vi "Section Names.vi"() -> (0 "Cluster":cluster{"Motion Settings":string}={"Motion Settings"="Motion Settings"})   [LabVIEW 2016, in "Hardware.lvlib" / "Motions.lvlib" / "Motions Configuration.lvclass"]
uses:
  <userlib>/Common Components/Hardware/Abstract System/Motions/Motions Config/Motions Configuration.lvclass
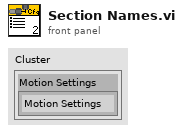
[diagram p1: front panel]
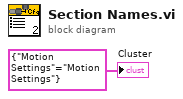
[diagram p0: block diagram]
diagram:
  "Cluster" <- cluster{"Motion Settings":string} {"Motion Settings"="Motion Settings"} ("Cluster")
